vi "Rename LLBs in XML File.vi"(7 "template base name":string, 8 "error in":errorcluster, 9 "xml name":string, 10 "CD name":string, 11 "custom device path":path) -> (0 "error out":errorcluster, 3 "custom device path out":path)   [LabVIEW 2020, in "Template Tool.lvlib"]
uses:
  Template Tool.lvlib
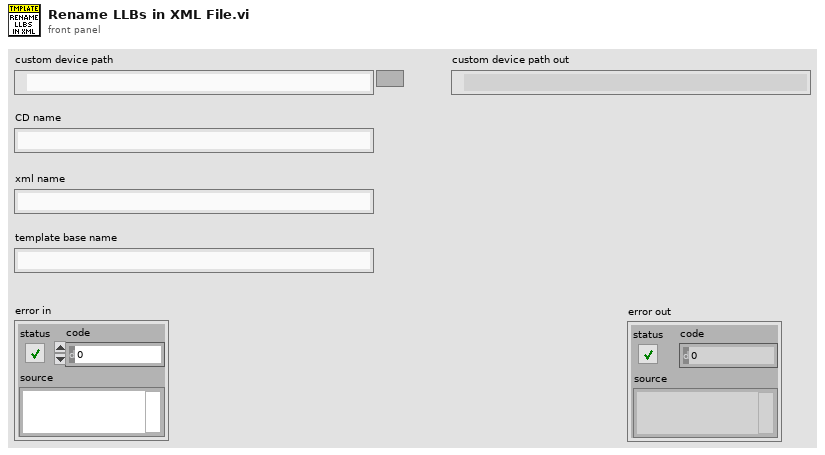
[diagram p1: front panel]
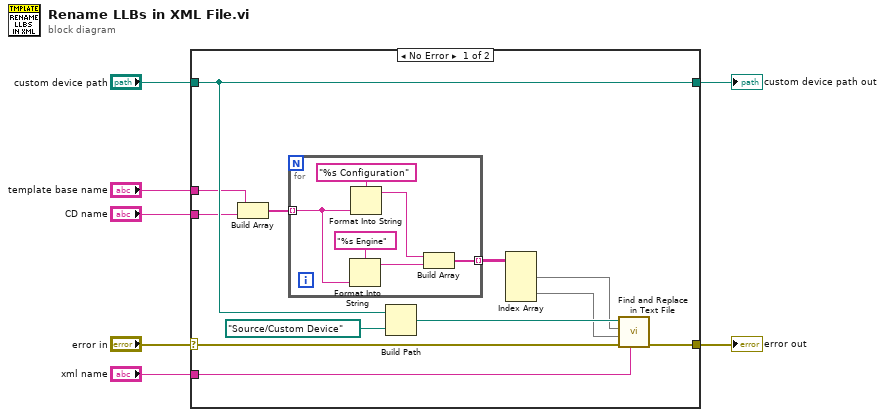
[diagram p0: block diagram]
diagram:
  n1 = case shown="No Error" "error in" {
    selector: "error in" -> [w18 w26]
    tunnel: "custom device path" -> [w17 w27]
    tunnel: [w16 w26] -> w7
    tunnel: [w17 w27] -> w4
    tunnel: "CD name" -> [w12 _]
    tunnel: "xml name" -> [w14 _]
    tunnel: "template base name" -> [w13 _]
    frame No Error {
      n2 = Build Array(w13, w12) -> (w11:string[])
      n3 = for {
        tunnel: [w25] -> w10 mode=indexing
        tunnel: w11 -> [w20] mode=indexing
        n4 = Format Into String(format string="%s Engine" ("string"), w20) -> (resulting string=w22:string)  [unwired: 2 in, 1 out]
        n5 = Format Into String(format string="%s Configuration" ("string"), w20) -> (resulting string=w24:string)  [unwired: 2 in, 1 out]
        n6 = Build Array(w24, w22) -> (w25:string[])
      }
      n7 = Build Path(base path=w17, name or relative path=path "Source/Custom Device") -> (appended path=w15:path)
      n8 = Index Array(array=w10) -> (element #1=w8:string[], element #2=w9:string[])  [unwired: 4 in]
      n9 = call "Find and Replace in Text File.vi"("file name"=w14, "error in"=w18, "replace array"=w9, "find array"=w8, "folder path"=w15) -> ("error out"=w16:errorcluster)  [unwired: 5 in, 1 out]
    }
    frame Error {
    }
  }
  "error out" <- w7
  "custom device path out" <- w4
